vi "PiezoStop.vi"(8 "error in (no error)":errorcluster caption="entrée d'erreur") -> (0 "error out":errorcluster caption="sortie d'erreur")   [LabVIEW 2009]
uses:
  Controls/PIEZO.COMMAND.ctl
  Controls/PIEZO.COMMANDBASIC.ctl
  Controls/PIEZO.WAVE.ctl
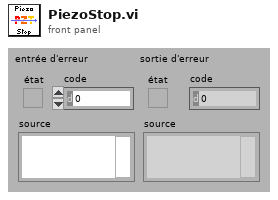
[diagram p1: front panel]
types:
  T1 = typedef "PIEZO.COMMAND.ctl" = cluster{"Command":T2, "WAVE":T3}
  T2 = typedef "PIEZO.COMMANDBASIC.ctl" = enum16{"RUN", "STOP", "QUIT"}
  T3 = typedef "PIEZO.WAVE.ctl" = cluster{"Speed":dbl[unit], "Stiffness (0.95)":dbl, "Linear Stroke":dbl[unit], "Delay":dbl[unit]}
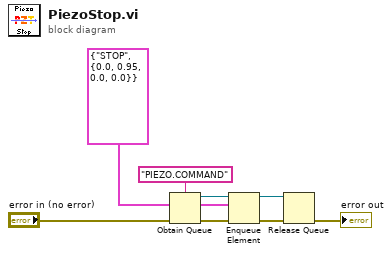
[diagram p0: block diagram]
diagram:
  w1 = T1 {"Command"=enum."STOP", "WAVE"={"Speed"=0.0, "Stiffness (0.95)"=0.95, "Linear Stroke"=0.0, "Delay"=0.0}} ("COMMAND")
  n1 = Obtain Queue(name (unnamed)="PIEZO.COMMAND" ("nom (aucun)"), element data type=w1, error in (no error)="error in (no error)") -> (queue out=w6:refnum<queue>, error out=w7:errorcluster)  [unwired: 2 in, 1 out]
  n2 = Enqueue Element(queue=w6, element=w1, error in (no error)=w7) -> (queue out=w5:refnum<queue>, error out=w4:errorcluster)  [unwired: 1 in, 1 out]
  n3 = Release Queue(queue=w5, error in (no error)=w4) -> (error out=→"error out":errorcluster)  [unwired: 1 in, 2 out]
